vi "Check Stop Acquisition.vi"(8 "Error In":errorcluster, 11 "Queue in":refnum<queue>) -> (0 "Error Out":errorcluster, 1 "Stop?":bool, 3 "Queue out":refnum<queue>)   [LabVIEW 2019]
uses:
  Controls/DAQ States.ctl
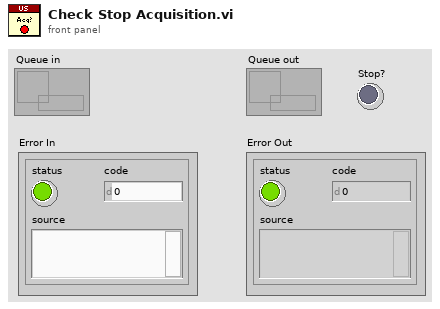
[diagram p1: front panel]
types:
  T1 = typedef "DAQ States.ctl" = enum16{"Initialize", "Idle", "Set Horizontal", "Set Vertical", "Set Trigger", "Set Display", "Acquire", "Analyze", "Set Switch", "Shutdown", "Quit"}
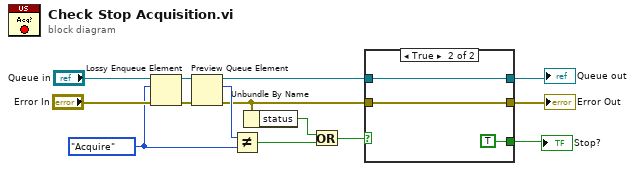
[diagram p0: block diagram]
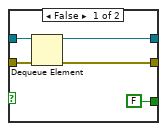
[diagram p2: hidden frame]
diagram:
  w9 = DAQ_States."Acquire" ("element")
  n1 = Lossy Enqueue Element(queue="Queue in", element=w9, error in (no error)="Error In") -> (queue out=w11:refnum<queue>, error out=w12:errorcluster)  [unwired: 2 out]
  n2 = Preview Queue Element(queue=w11, error in (no error)=w12) -> (queue out=w8:refnum<queue>, element=w10:T1, error out=w4:errorcluster)  [unwired: 1 in, 1 out]
  n3 = Not Equal?(x=w10, y=w9) -> (x != y?=w3:bool)
  n4 = Unbundle By Name(w4) -> ("status"=w1:bool)
  n5 = Or(x=w1, y=w3) -> (x .or. y?=w2:bool)
  n6 = case shown="True" w2 {
    tunnel: w8 -> [w19 w22]
    tunnel: w4 -> [w18 w21]
    tunnel: [w17 w22] -> w6
    tunnel: [w16 w21] -> w7
    tunnel: [FALSE ("status") TRUE ("status")] -> w5
    frame False {
      n7 = Dequeue Element(queue=w19, error in (no error)=w18) -> (queue out=w17:refnum<queue>, error out=w16:errorcluster)  [unwired: 1 in, 2 out]
    }
    frame True {
    }
  }
  "Error Out" <- w7
  "Stop?" <- w5
  "Queue out" <- w6
